vi "setQuackBehavior.vi"(8 "error in (no error)":errorcluster, 10 "QuackBehavior.lvclass":refnum<class "QuackBehavior.lvclass">, 11 "Duck in":refnum<class "Duck.lvclass">) -> (0 "error out":errorcluster, 3 "Duck out":refnum<class "Duck.lvclass">)   [LabVIEW 2013, in "Duck.lvclass"]
uses:
  Duck.lvclass
  QuackBehavior/QuackBehavior.lvclass
  Duck.lvclass/Duck.ctl
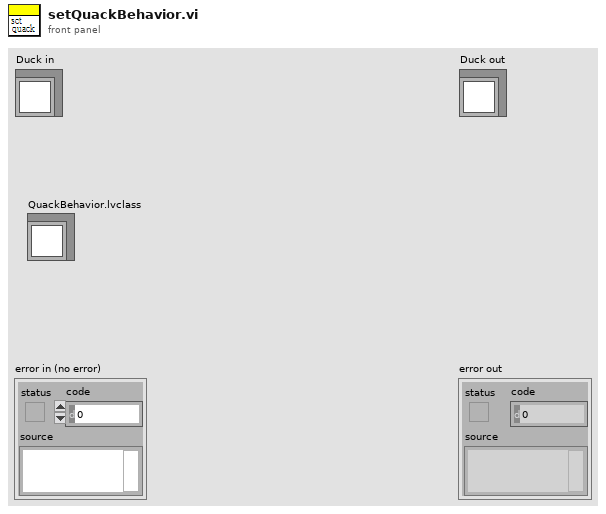
[diagram p1: front panel]
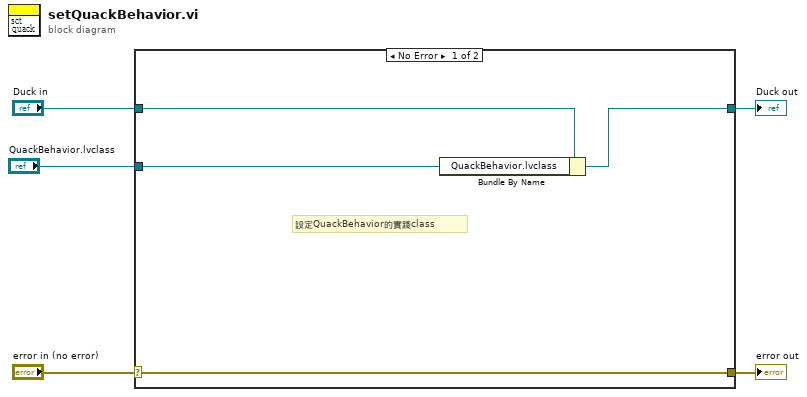
[diagram p0: block diagram]
diagram:
  n1 = case shown="No Error" "error in (no error)" {
    selector: "error in (no error)" -> [w9 w11]
    tunnel: [w9 w11] -> w4
    tunnel: [w7 w10] -> w2
    tunnel: "Duck in" -> [w8 w10]
    tunnel: "QuackBehavior.lvclass" -> [w6 _]
    frame No Error {
      # "設定QuackBehavior的實踐class"
      n2 = Bundle By Name(cluster=w8, "QuackBehavior.lvclass"=w6) -> (w7:refnum<class "Duck.lvclass">)
    }
    frame Error {
    }
  }
  "error out" <- w4
  "Duck out" <- w2
